vi "ActDriveStraightCalcError-Alt2.vi"(10 "Dist (ft)":dbl, 11 "FirstTime":bool) -> (3 "Error":dbl)   [LabVIEW 2020]
uses:
  DriveSystem/DriveGlobals.vi
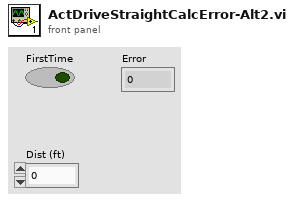
[diagram p1: front panel]
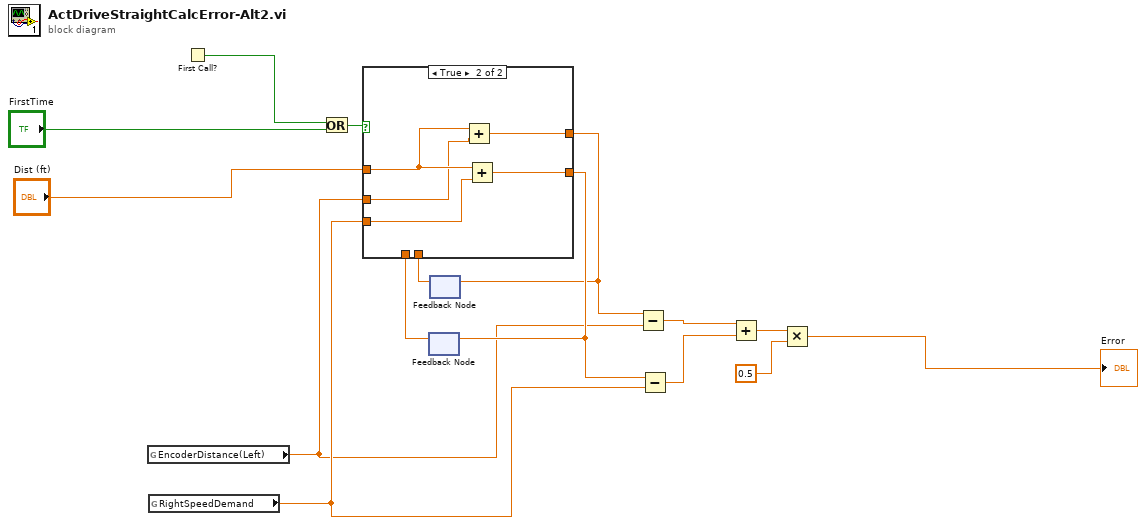
[diagram p0: block diagram]
diagram:
  n1 = global read "DriveGlobals.vi" "EncoderDistance(Left)"() -> (w5:dbl)
  n2 = global read "DriveGlobals.vi" "RightSpeedDemand"() -> (w6:dbl)
  n3 = First Call?() -> (First Call?: T/F=w1:bool)
  n4 = Or(x=w1, y="FirstTime") -> (x .or. y?=w3:bool)
  n5 = feedback #1() -> (w10:dbl)  [unwired: 1 in]
  n6 = feedback #2() -> (w9:dbl)  [unwired: 1 in]
  n7 = case shown="True" w3 {
    tunnel: "Dist (ft)" -> [_ w22]
    tunnel: w5 -> [_ w21]
    tunnel: w6 -> [_ w20]
    tunnel: [w17 w19] -> w7
    tunnel: [w16 w18] -> w8
    tunnel: w9 -> [w17 _]
    tunnel: w10 -> [w16 _]
    frame False {
    }
    frame True {
      n8 = Add(x=w22, y=w21) -> (x+y=w19:dbl)
      n9 = Add(x=w22, y=w20) -> (x+y=w18:dbl)
    }
  }
  n10 = feedback-in #1(w8) -> ()
  n11 = feedback-in #2(w7) -> ()
  n12 = Subtract(x=w7, y=w5) -> (x-y=w11:dbl)
  n13 = Subtract(x=w8, y=w6) -> (x-y=w12:dbl)
  n14 = Add(x=w11, y=w12) -> (x+y=w13:dbl)
  n15 = Multiply(x=w13, y=0.5) -> (x*y=→"Error":dbl)
